vi "CST_CtrlRefShifter.vi"() -> (0 "App Ctrl Refs":T1)   [LabVIEW 2010]
uses:
  Controls/Shift Registers/TYP_CtrlRefShifter.ctl
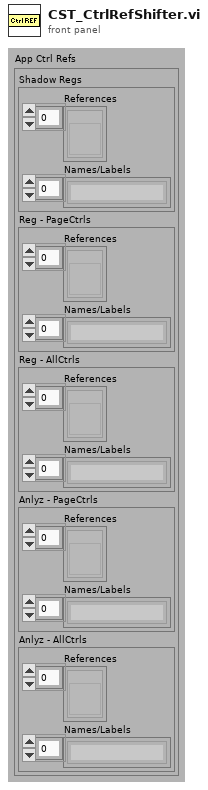
[diagram p1: front panel]
types:
  T1 = typedef "TYP_CtrlRefShifter.ctl" = cluster{"Shadow Regs":cluster{"References":refnum<vi>[], "Names/Labels":string[]}, "Reg - PageCtrls":cluster{"References":refnum<vi>[], "Names/Labels":string[]}, "Reg - AllCtrls":cluster{"References":refnum<vi>[], "Names/Labels":string[]}, "Anlyz - PageCtrls":cluster{"References":refnum<vi>[], "Names/Labels":string[]}, "Anlyz - AllCtrls":cluster{"References":refnum<vi>[], "Names/Labels":string[]}}
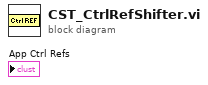
[diagram p0: block diagram]
diagram:
